vi "[Global]PatternMatchNumber.vi"() -> ()   [LabVIEW 2015]
panel:
  in  "PatternMatchNumber":i32=20
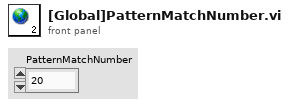
[diagram p1: front panel]
diagram:
